vi "Report Unsupported Enumerated Argument Value.vi"(9 "Supported Values":string[](array[string]), 10 "Unsupported Value":string, 11 "Argument":string) -> (0 "error out":errorcluster)   [LabVIEW 2014, in "RunVIAnalyzer.lvclass"]
uses:
  RunVIAnalyzer.lvclass
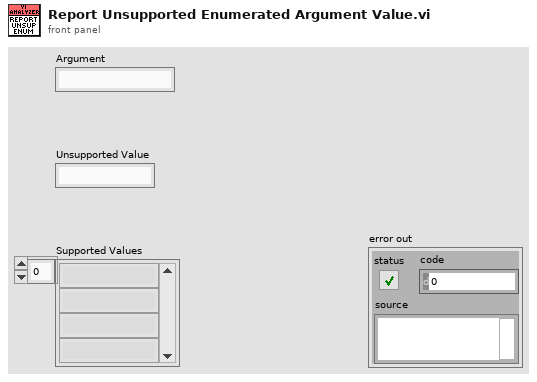
[diagram p1: front panel]
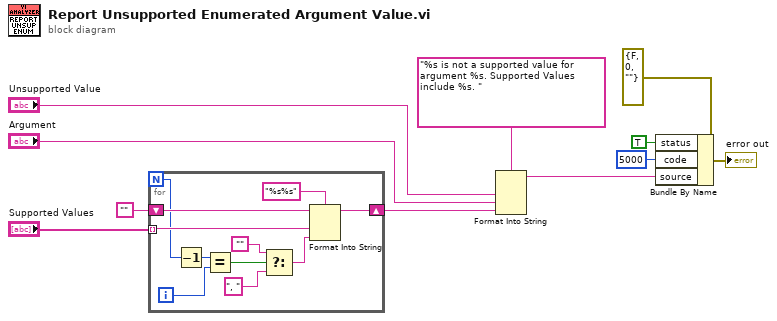
[diagram p0: block diagram]
diagram:
  n1 = for {
    N -> [w18]
    tunnel: "Supported Values" -> [w20] mode=indexing
    shift-right: [w21] -> w3
    shift-left: "" -> [w22]
    i -> [w17]
    n2 = Decrement(x=w18) -> (x-1=w13:i32)
    n3 = Equal?(x=w13, y=w17) -> (x = y?=w16:bool)
    n4 = Select(t="", s=w16, f=", ") -> (s? t:f=w14:string)
    n5 = Format Into String(format string="%s%s", initial string=w22, w20, w14) -> (resulting string=w21:string)  [unwired: 1 in, 1 out]
  }
  n6 = Format Into String(format string="%s is not a supported value for argument %s. Supported Values include %s. ", "Unsupported Value", "Argument", w3) -> (resulting string=w7:string)  [unwired: 2 in, 1 out]
  n7 = Bundle By Name(cluster=errorcluster {"status"=FALSE, "code"=0, "source"=""} ("error out"), "status"=TRUE, "code"=5000, "source"=w7) -> (→"error out":errorcluster)
